vi "signal_conditioning_diag.vi"(8 "averaging time":dbl=0.1 format="%0.2p", 9 "dt":dbl, 10 "t_LD":dbl[](array[numeric]), 11 "all rows":dbl[][](array[numeric]) format="%0.3f") -> (2 "Dc offset":waveform(dbl)(graph), 3 "Offset removed":cluster{"xi used":dbl[], "yi":dbl[]}(graph))   [LabVIEW 2015]
uses:
  <vilib>/measure/madcrms.llb/Averaged DC-RMS for 1 Chan.vi
  <vilib>/Waveform/WDTOps.llb/WDT Get Waveform Time Array DBL.vi
  <vilib>/measure/NI_MAPro.lvlib
  <vilib>/gmath/NI_Gmath.lvlib
panel:
  out "LD Signal":waveform(dbl)(graph)
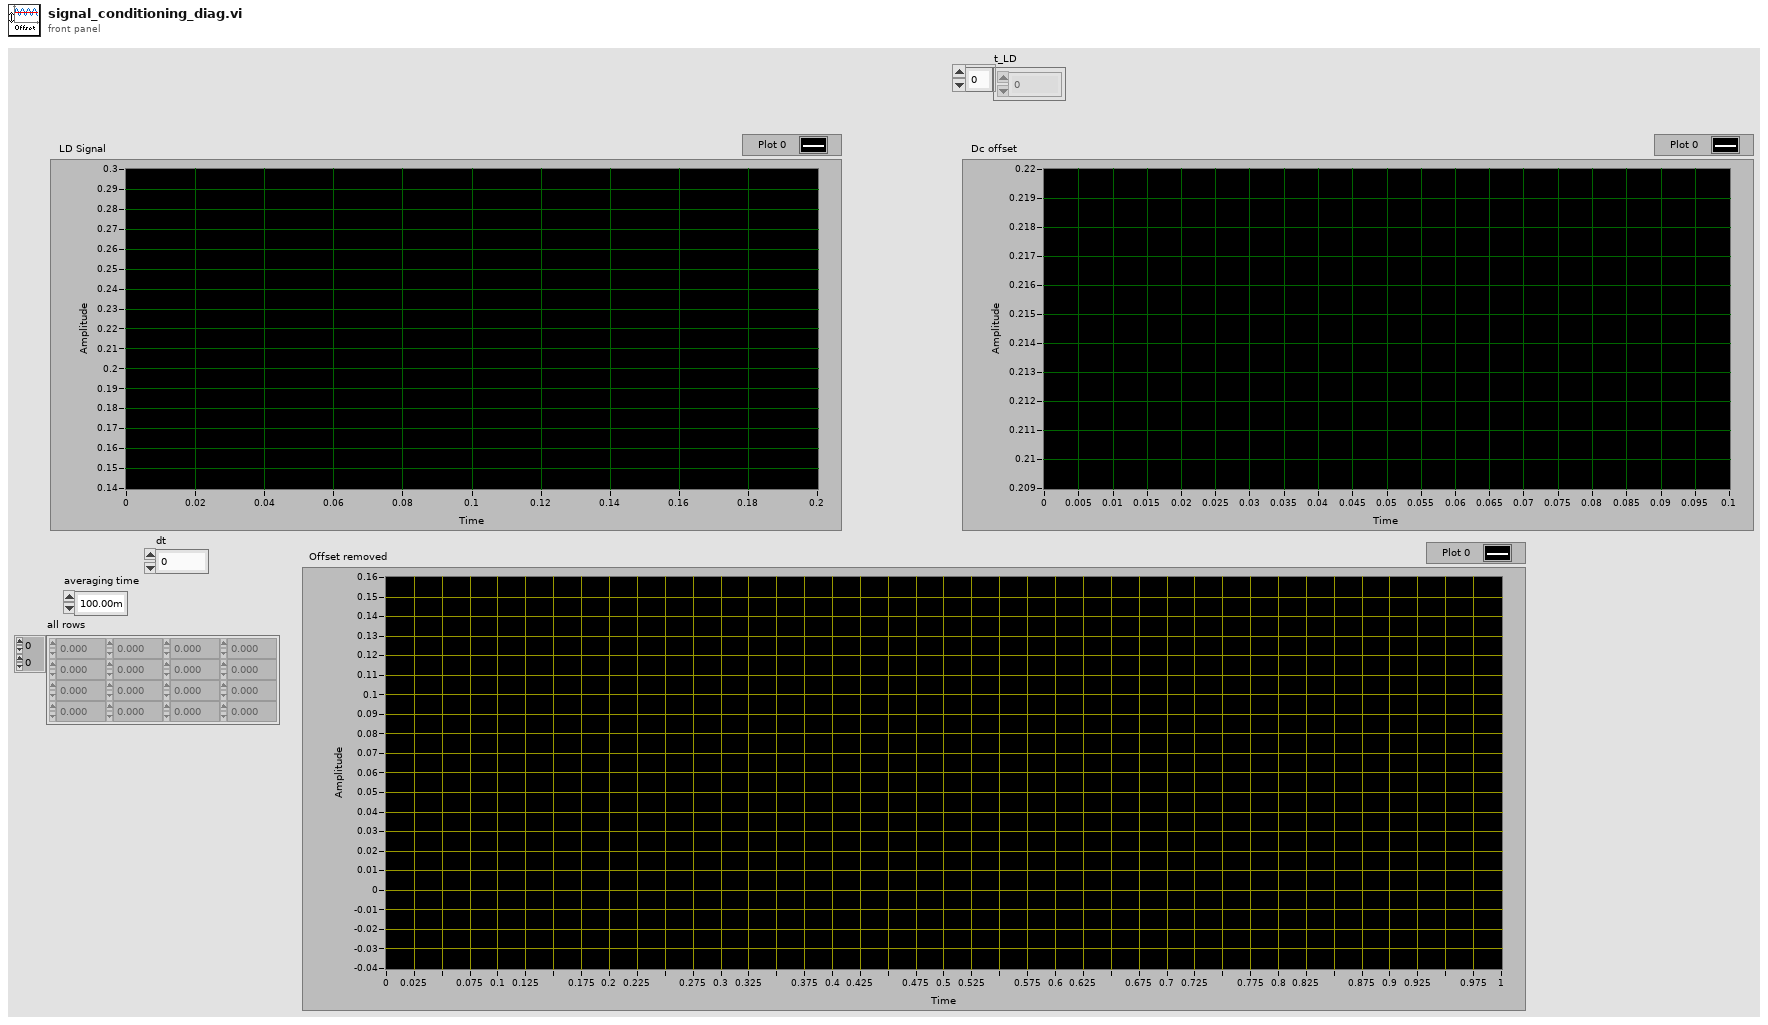
[diagram p1: front panel]
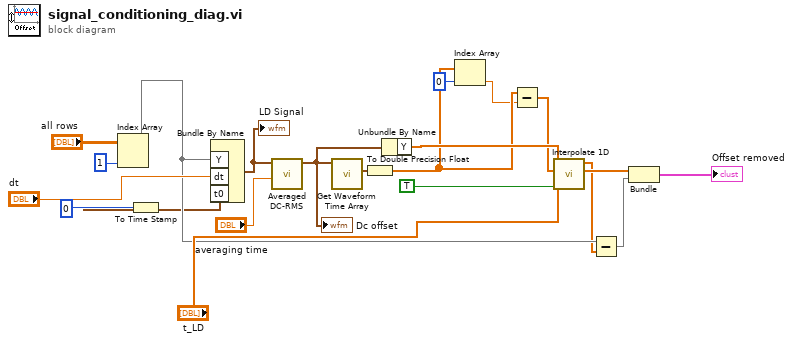
[diagram p0: block diagram]
diagram:
  n1 = Index Array(array="all rows", index (col)=1 ("disabled index (col)")) -> (element=w14:dbl[])  [unwired: 1 in]
  n2 = To Time Stamp(1:0) -> (0:w5:timestamp)
  n3 = Bundle By Name("Y"=w14, "dt"="dt", "t0"=w5) -> (w19:waveform(dbl))  [unwired: 1 in]
  "LD Signal" <- w19
  n4 = call-poly <vilib>:"Averaged DC-RMS.vi"("averaging time"="averaging time", "signal in"=w19) -> ("DC value waveform"=w16:waveform(dbl))  [unwired: 5 in, 4 out]
  "Dc offset" <- w16
  n5 = call-poly <vilib>:"Get Waveform Time Array.vi"("waveform in"=w16) -> ("X array"=w17:timestamp[])  [unwired: 9 in, 1 out]
  n6 = To Double Precision Float(number=w17) -> (double precision float=w3:dbl[])
  n7 = Unbundle By Name(w16) -> ("Y"=w15:dbl[])
  n8 = Index Array(array=w3, index=0) -> (element=w2:dbl)
  n9 = Subtract(x=w3, y=w2) -> (x-y=w1:dbl[])
  n10 = call <vilib>:"Interpolate 1D.vi"("X is monotonic"=TRUE, "xi"="t_LD", "X"=w1, "Y"=w15) -> ("xi used"=w11:dbl[], "yi"=w10:dbl[])  [unwired: 5 in, 1 out]
  n11 = Subtract(x=w14, y=w10) -> (x-y=w13:dbl[])
  n12 = Bundle("xi used"=w11, w13) -> (→"Offset removed":cluster{"xi used":dbl[], dbl[]})  [unwired: 1 in]
